vi "AMX-电源头正面标签凹凸检测参数读取.vi"(7 "error in (no error)":errorcluster caption="错误输入（无错误）", 10 "基路径":path) -> (0 "error out":errorcluster caption="错误输出", 2 "UI电源线正面凹凸参数":T1={"Min Radius"=7.0, "Max Radius"=11.0, "Max Number"=11.0}, 3 "UI电源线正面漏线基础参数":T2={"IsNorImage"=TRUE, "Exposure Values"=100289, "ImagePath"=path "C:/Users/hedongpo/Desktop/514-hdp/Alignment Assemble System/Test Picture/B/3.bmp"} caption="参数界面" {"Exposure Values" scale=0.0..200000.0})   [LabVIEW 2017]
uses:
  <vilib>/Utility/xml.llb/Read From XML File(string).vi
  Global System.vi
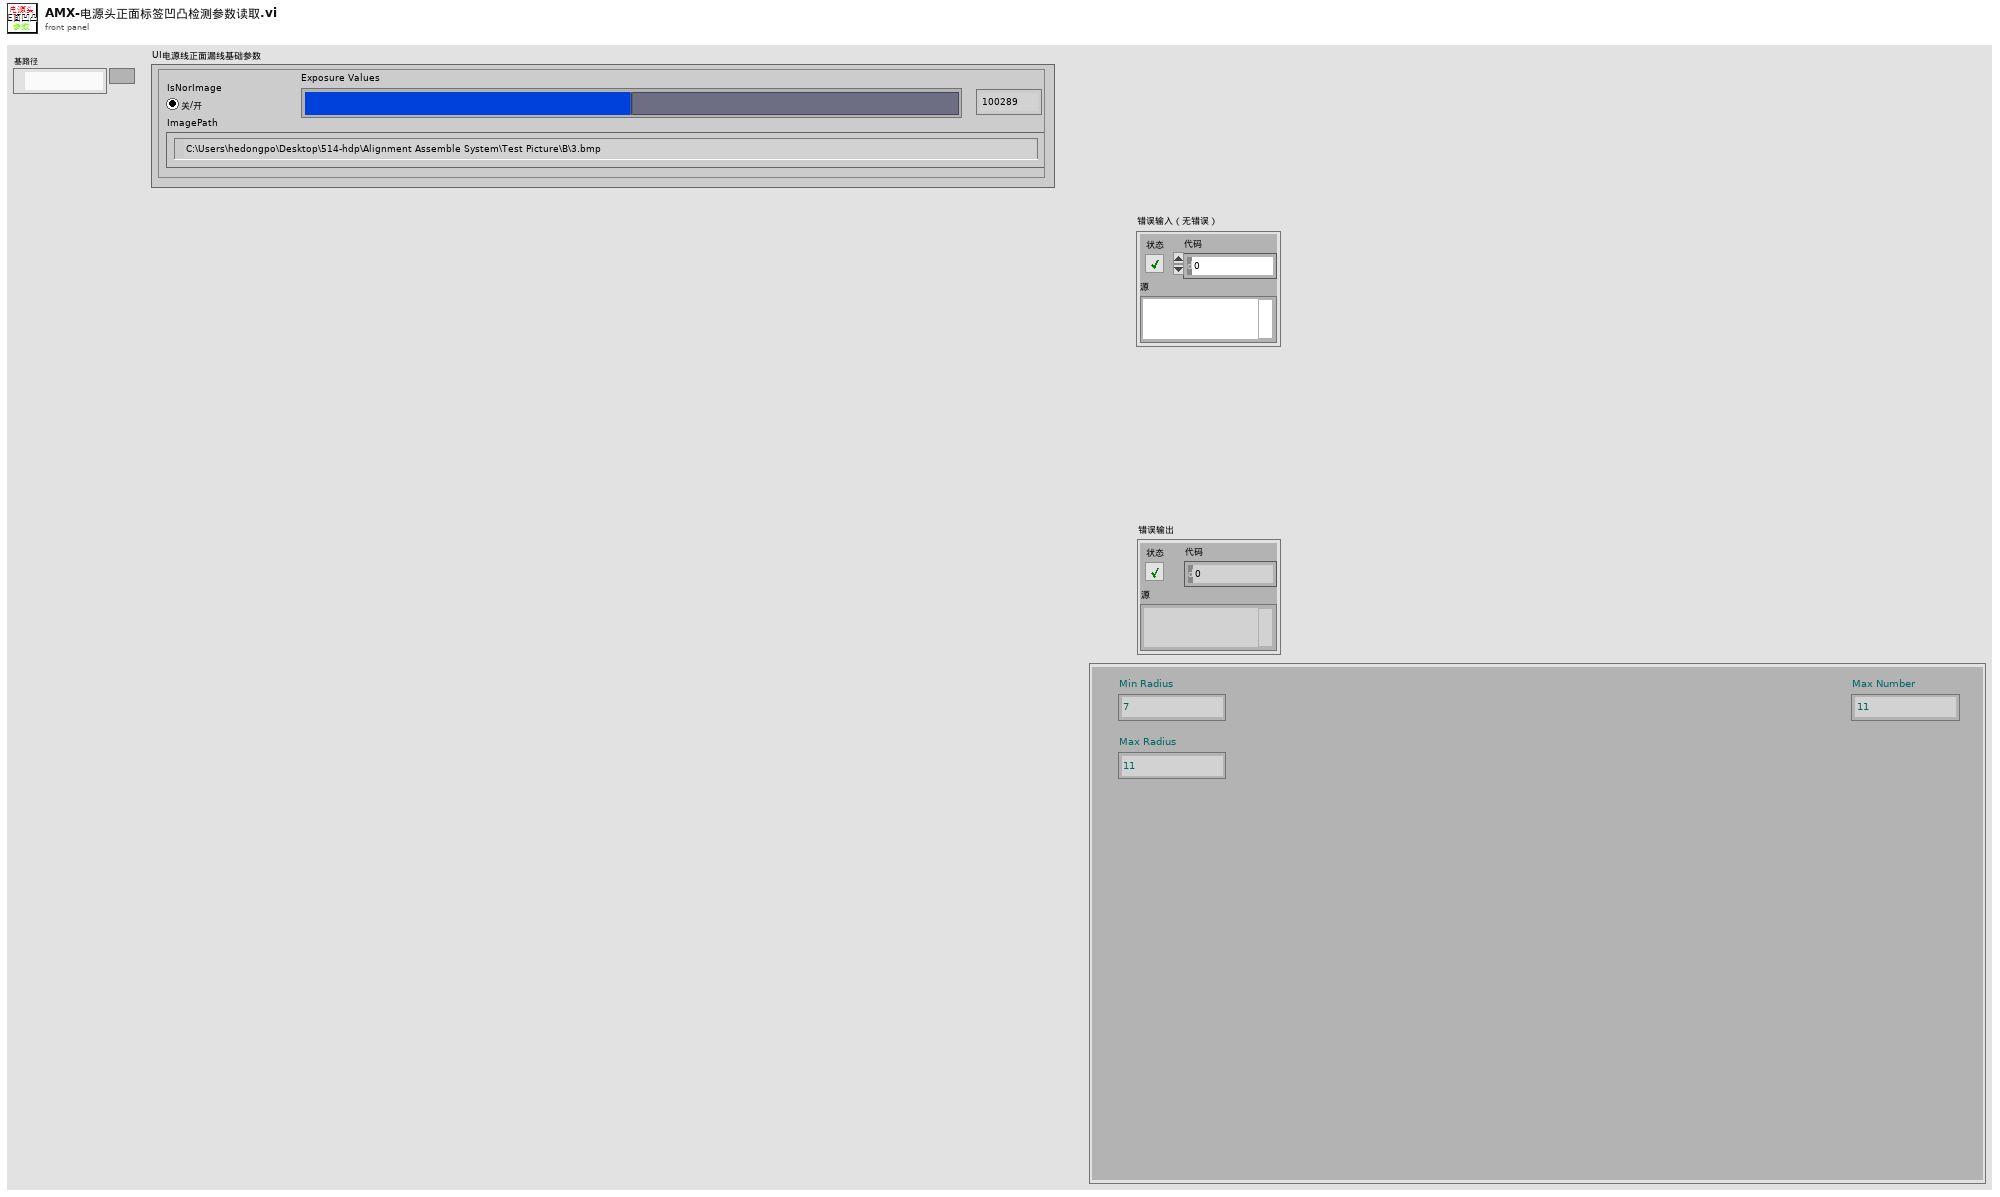
[diagram p1: front panel]
types:
  T1 = cluster{"Min Radius":sgl, "Max Radius":sgl, "Max Number":sgl}
  T2 = cluster{"IsNorImage":bool, "Exposure Values":u32, "ImagePath":path}
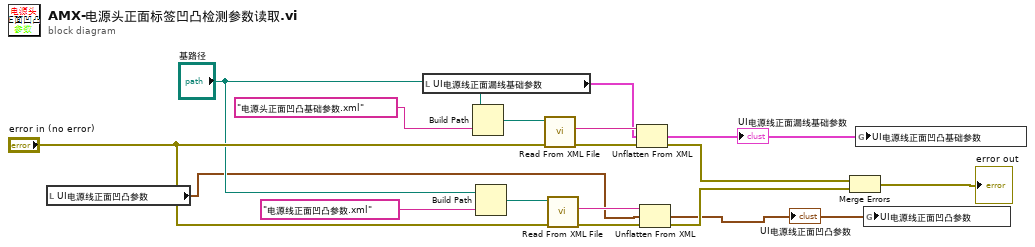
[diagram p0: block diagram]
diagram:
  n1 = local read "UI电源线正面凹凸参数"() -> (w2:T1)
  n2 = local read "UI电源线正面漏线基础参数"() -> (w6:T2)
  n3 = Build Path(base path="基路径", name or relative path="电源头正面凹凸基础参数.xml" ("名称或相对路径")) -> (appended path=w17:path)
  n4 = Build Path(base path="基路径", name or relative path="电源线正面凹凸参数.xml" ("名称或相对路径")) -> (appended path=w14:path)
  n5 = call-poly <vilib>:"Read From XML File.vi"("error in (no error)"="error in (no error)", "XML File Path"=w17) -> ("error out"=w12:errorcluster, "XML Elements"=w16:string)  [unwired: 7 in, 1 out]
  n6 = call-poly <vilib>:"Read From XML File.vi"("error in (no error)"="error in (no error)", "XML File Path"=w14) -> ("error out"=w10:errorcluster, "XML Elements"=w15:string)  [unwired: 7 in, 1 out]
  n7 = Unflatten From XML(xml string=w16, type=w6, error in (no error)=w12) -> (value=w3:T2, error out=w11:errorcluster)
  "UI电源线正面漏线基础参数" <- w3
  n8 = Unflatten From XML(xml string=w15, type=w2, error in (no error)=w10) -> (value=w1:T1, error out=w9:errorcluster)
  "UI电源线正面凹凸参数" <- w1
  n9 = Merge Errors(w11, w9) -> (→"error out":errorcluster)
  n10 = global write "Global System.vi" "UI电源线正面凹凸基础参数"(w3) -> ()
  n11 = global write "Global System.vi" "UI电源线正面凹凸参数"(w1) -> ()
